vi "mod_Demodulate AM.vi"   [LabVIEW 2020, in "niAMT.lvlib"]
uses:
  <vilib>/addons/Modulation/niAMT.lvlib
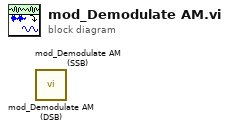
[diagram p0: block diagram]
diagram:
  n1 = call <vilib>:"mod_Demodulate AM (DSB).vi"() -> ()  [unwired: 13 in, 3 out]
  n2 = call <vilib>:"mod_Demodulate AM (SSB).vi"() -> ()  [unwired: 12 in, 4 out]
